vi "support_locateConfigDir.vi"(8 "error in (no error)":errorcluster) -> (0 "error IO":errorcluster, 3 "Config path":path)   [LabVIEW 2015]
doc: "locates <b>Config</b> folder\n---------------------------------------------------------------\nAuthor: Dang Lam\nEmail: danglamtd@gmail.com"
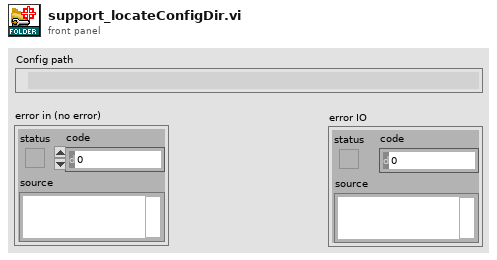
[diagram p1: front panel]
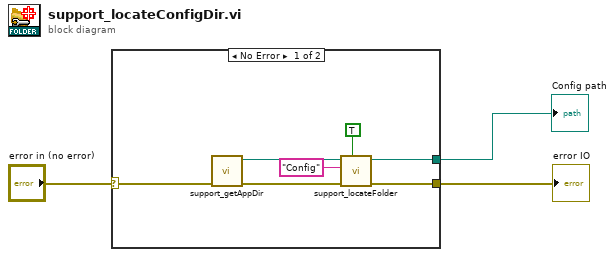
[diagram p0: block diagram]
diagram:
  n1 = case shown="No Error" "error in (no error)" {
    selector: "error in (no error)" -> [w10 w11]
    tunnel: [w8 w11] -> w2
    tunnel: [w4 _] -> w1
    frame No Error {
      n2 = call "support_getAppDir.vi"("error in (no error)"=w10) -> ("error out"=w9:errorcluster, "App.Dir"=w7:path)  [unwired: 9 in]
      n3 = call "support_locateFolder.vi"("create if not found?"=TRUE, "error in (no error)"=w9, "Folder"="Config" ("folder"), "Root"=w7) -> ("error IO"=w8:errorcluster, "path"=w4:path)  [unwired: 5 in, 1 out]
    }
    frame Error {
    }
  }
  "error IO" <- w2
  "Config path" <- w1
